vi "Contiguous Check.vi"(8 "error in (no error)":errorcluster, 11 "channel offsets in":u64[](array[numeric])) -> (0 "error out":errorcluster, 2 "contiguous?":bool, 3 "channel offsets out":u64[](array[numeric]))   [LabVIEW 2017, in "DSF Engine.lvlib" / "VeriStand DSF.lvclass"]
uses:
  VeriStand DSF.lvclass
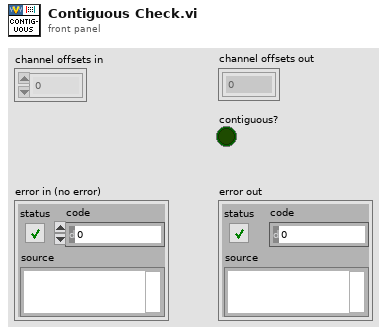
[diagram p1: front panel]
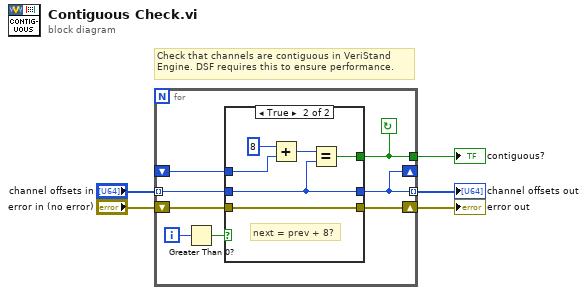
[diagram p0: block diagram]
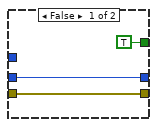
[diagram p2: hidden frame]
diagram:
  # "Check that channels are contiguous in VeriStand Engine. DSF requires this to ensure performance."
  n1 = for {
    tunnel: "channel offsets in" -> [w11] mode=indexing
    shift-right: [w8] -> w2
    shift-left: "error in (no error)" -> [w10]
    shift-right: [w6] -> _
    shift-left: _ -> [w9]
    tunnel: [w7] -> w3
    tunnel: [w6] -> w4 mode=indexing
    i -> [w13]
    stop <- w7 continue-if-true
    n2 = Greater Than 0?(x=w13) -> (x > 0?=w12:bool)
    n3 = case shown="True" w12 {
      tunnel: w11 -> [w15 w18]
      tunnel: w10 -> [w16 w17]
      tunnel: w9 -> [_ w22]
      tunnel: [w16 w17] -> w8
      tunnel: [TRUE w19] -> w7
      tunnel: [w15 w18] -> w6
      frame False {
      }
      frame True {
        # "next = prev + 8?"
        n4 = Add(x=u64 8 ("y"), y=w22) -> (x+y=w20:u64)
        n5 = Equal?(x=w20, y=w18) -> (x = y?=w19:bool)
      }
    }
  }
  "channel offsets out" <- w4
  "contiguous?" <- w3
  "error out" <- w2
